vi "Add LVCI to Config.vi"() -> ()   [LabVIEW 2014]
uses:
  <vilib>/Utility/sysdir.llb/System Directory Type.ctl
  <vilib>/Utility/config.llb/Read Key (String).vi
  <vilib>/Utility/config.llb/Write Key (String).vi
  <vilib>/Utility/config.llb/NI_LVConfig.lvlib
  <vilib>/httpClient/LabVIEWHTTPClient.lvlib
panel:
  in  "OK Button":bool
  in  "LabVIEW Machine Name":string
  in  "LabVIEW Machine Port":u32
  in  "Path to Jobber":path
  in  "LabVIEW Path":path
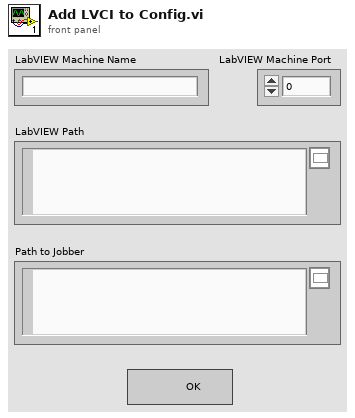
[diagram p1: front panel]
types:
  T1 = typedef "System Directory Type.ctl" = i32
  T2 = typedef "NI_LVConfig.lvlib/Config Data RefNum.ctl" = refnum<k1>
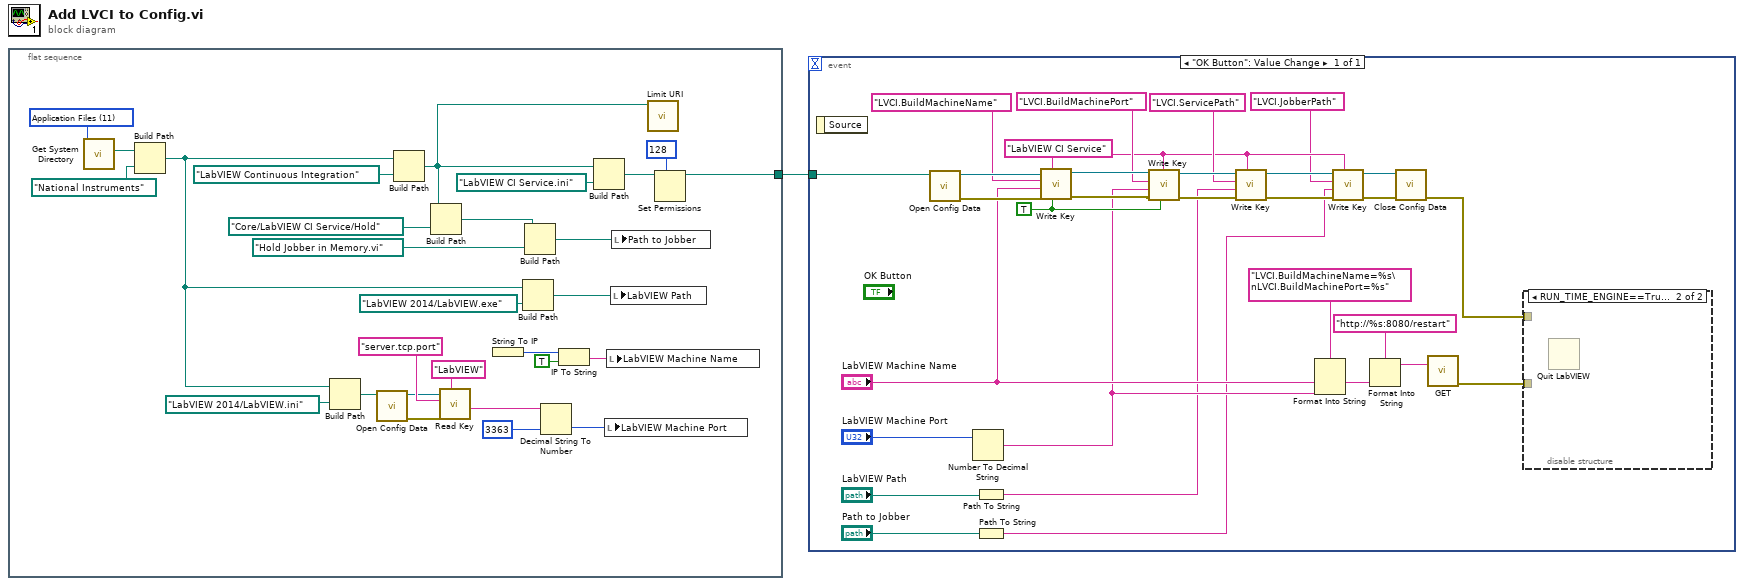
[diagram p0: block diagram]
diagram:
  n1 = flat-sequence {
    tunnel: [w27] -> w1
    frame #0 {
      w13 = T1 11 items=["User Home"=0, "User Desktop"=1, "User Documents"=2, "User Application Data"=3, "User Preferences"=4, "User Temporary"=5, "Public Documents"=6, "Public Application Data"=7, "Public Preferences"=8, "Public Cache"=13, "System Core Libraries"=9, "System Installed Libraries"=10, "Application Files"=11, "Boot Volume Root"=12] ("system directory type")
      n2 = call <vilib>:"Get System Directory.vi"("system directory type"=w13) -> ("system directory"=w7:path)  [unwired: 10 in]
      n3 = Build Path(base path=w7, name or relative path=path "National Instruments" ("appended path")) -> (appended path=w3:path)
      n4 = Build Path(base path=w3, name or relative path=path "LabVIEW 2014/LabVIEW.ini" ("appended path")) -> (appended path=w6:path)
      n5 = call <vilib>:"Open Config Data.vi"("configuration file path"=w6) -> ("error out"=w11:errorcluster, "refnum"=w9:T2)  [unwired: 8 in, 1 out]
      n6 = Build Path(base path=w3, name or relative path=path "LabVIEW Continuous Integration") -> (appended path=w26:path)
      n7 = Build Path(base path=w26, name or relative path=path "Core/LabVIEW CI Service/Hold") -> (appended path=w25:path)
      n8 = call-poly <vilib>:"Read Key.vi"("section"="LabVIEW", "error in (no error)"=w11, "key"="server.tcp.port" ("default value"), "refnum"=w9) -> ("value"=w8:string)  [unwired: 4 in, 3 out]
      n9 = String To IP() -> (0:w29:u32)  [unwired: 1 in]
      n10 = Build Path(base path=w3, name or relative path=path "LabVIEW 2014/LabVIEW.exe" ("appended path")) -> (appended path=w5:path)
      n11 = Build Path(base path=w25, name or relative path=path "Hold Jobber in Memory.vi") -> (appended path=w21:path)
      n12 = Decimal String To Number(string=w8, default (0L)=u32 3363 ("LabVIEW Machine Port")) -> (number=w22:u32)  [unwired: 1 in, 1 out]
      n13 = IP To String(1:TRUE ("dot notation? (F)"), 2:w29) -> (0:w24:string)
      n14 = Build Path(base path=w26, name or relative path=path "LabVIEW CI Service.ini") -> (appended path=w17:path)
      n15 = local write "LabVIEW Machine Port"(w22) -> ()
      n16 = local write "LabVIEW Machine Name"(w24) -> ()
      n17 = local write "LabVIEW Path"(w5) -> ()
      n18 = local write "Path to Jobber"(w21) -> ()
      n19 = call "Limit URI.vi"("base path"=w26) -> ()  [unwired: 10 in, 1 out]
      n20 = Set Permissions(7:i16 128 ("permissions"), 11:w17) -> (3:w27:path)  [unwired: 3 in, 1 out]
    }
  }
  n21 = event shown="[0] \"OK Button\": Value Change" {
    selector: _ -> [_]
    dyn-events: _ -> [_]
    timeout: _ -> [_]
    tunnel: w1 -> [w57]
    event "OK Button": Value Change {
      w50 = TRUE ("write raw string? (F)")
      w40 = "LabVIEW CI Service" ("section")
      n22 = event-data() -> ()  [unwired: 1 in, 1 out]
      n23 = call <vilib>:"Open Config Data.vi"("configuration file path"=w57) -> ("error out"=w51:errorcluster, "refnum"=w56:T2)  [unwired: 8 in, 1 out]
      n24 = Number To Decimal String(number="LabVIEW Machine Port") -> (decimal integer string=w36:string)  [unwired: 1 in]
      n25 = Path To String(path="LabVIEW Path") -> (string=w32:string)
      n26 = Path To String(path="Path to Jobber") -> (string=w34:string)
      n27 = call-poly <vilib>:"Write Key.vi"("write raw string? (F)"=w50, "section"=w40, "error in (no error)"=w51, "value"="LabVIEW Machine Name", "key"="LVCI.BuildMachineName", "refnum"=w56) -> ("error out"=w53:errorcluster, "refnum out"=w54:T2)  [unwired: 3 in, 1 out]
      n28 = call-poly <vilib>:"Write Key.vi"("write raw string? (F)"=w50, "section"=w40, "error in (no error)"=w53, "value"=w36, "key"="LVCI.BuildMachinePort", "refnum"=w54) -> ("error out"=w48:errorcluster, "refnum out"=w49:T2)  [unwired: 3 in, 1 out]
      n29 = call-poly <vilib>:"Write Key.vi"("section"=w40, "error in (no error)"=w48, "value"=w32, "key"="LVCI.ServicePath", "refnum"=w49) -> ("error out"=w42:errorcluster, "refnum out"=w44:T2)  [unwired: 4 in, 1 out]
      n30 = Format Into String(format string="LVCI.BuildMachineName=%s\nLVCI.BuildMachinePort=%s", "LabVIEW Machine Name", w36) -> ()  [unwired: 2 in, 2 out]
      n31 = call-poly <vilib>:"Write Key.vi"("section"=w40, "error in (no error)"=w42, "value"=w34, "key"="LVCI.JobberPath", "refnum"=w44) -> ("error out"=w41:errorcluster, "refnum out"=w43:T2)  [unwired: 4 in, 1 out]
      n32 = Format Into String(format string="http://%s:8080/restart", "LabVIEW Machine Name") -> (resulting string=w45:string)  [unwired: 2 in, 1 out]
      n33 = call <vilib>:"Close Config Data.vi"("error in (no error)"=w41, "refnum"=w43) -> ("error out"=w30:errorcluster)  [unwired: 8 in, 1 out]
      n34 = call <vilib>:"GET.vi"("url"=w45) -> ("error out"=w31:errorcluster)  [unwired: 11 in, 3 out]
      n35 = disable-structure shown="RUN_TIME_ENGINE==True" {
        disable-tunnel: w31 -> [_ _]
        disable-tunnel: w30 -> [_ _]
        frame condition #0 (active) {
        }
        frame condition #1 {
          n36 = Quit LabVIEW() -> ()  [unwired: 1 in]
        }
      }
    }
  }
